vi "Cleanup.vi"(8 "error in (no error)":errorcluster, 11 "TCP_Streamer in":refnum<class "TCP_Streamer_Publisher.lvclass">) -> (0 "error out":errorcluster, 3 "TCP_Streamer out":refnum<class "TCP_Streamer_Publisher.lvclass">)   [LabVIEW 2021, in "TCP_Streamer_Publisher.lvclass"]
uses:
  TCP_Streamer_Publisher.lvclass
  TCP_Streamer_Publisher.lvclass/TCP_Streamer_Publisher.ctl
  Typedef/State.ctl
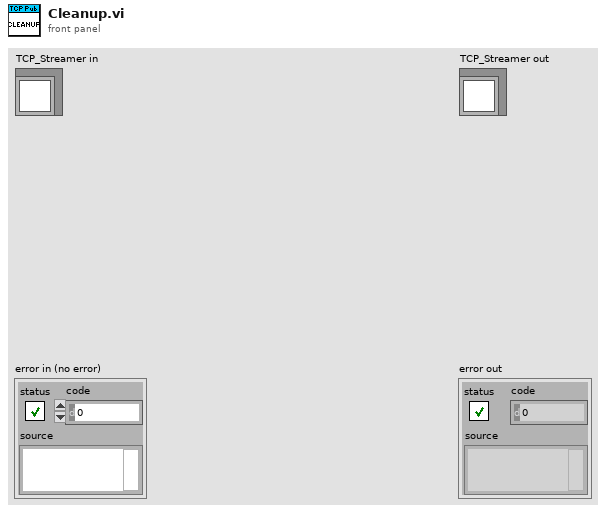
[diagram p1: front panel]
types:
  T1 = typedef "TCP_Streamer_Publisher.lvclass/State.ctl" = enum16{"Stopped", "Listening", "Ready for Data", "Ready to Send", "Sending"}
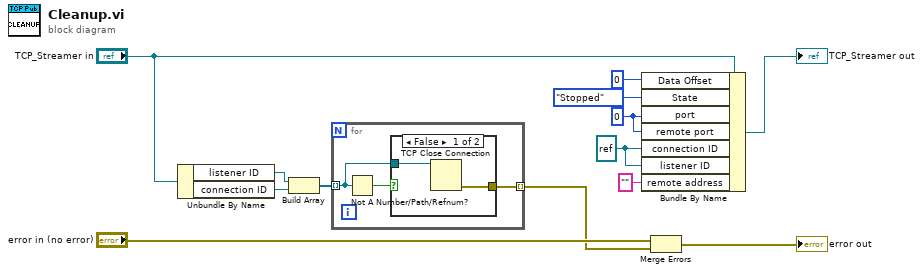
[diagram p0: block diagram]
diagram:
  w7 = refnum<k5> refnum ("connection ID")
  w8 = u16 0 ("port")
  n1 = Unbundle By Name("TCP_Streamer in") -> ("listener ID"=w12:refnum<k5>, "connection ID"=w13:refnum<k5>)
  n2 = Build Array(w12, w13) -> (w11:refnum<k5>[])
  n3 = for {
    tunnel: w11 -> [w15] mode=indexing
    tunnel: [w14] -> w3 mode=indexing
    n4 = Not A Number/Path/Refnum?(number/path/refnum=w15) -> (NaN/Path/Refnum?=w16:bool)
    n5 = case shown="False" w16 {
      tunnel: [w18 _] -> w14
      tunnel: w15 -> [w17 _]
      frame False {
        n6 = TCP Close Connection(connection ID=w17) -> (error out=w18:errorcluster)  [unwired: 2 in, 1 out]
      }
      frame True {
      }
    }
  }
  n7 = Bundle By Name(cluster="TCP_Streamer in", "Data Offset"=0, "State"=State."Stopped", "port"=w8, "remote port"=w8, "connection ID"=w7, "listener ID"=w7, "remote address"="") -> (→"TCP_Streamer out":refnum<class "TCP_Streamer_Publisher.lvclass">)
  n8 = Merge Errors("error in (no error)", w3) -> (→"error out":errorcluster)
